vi "module-05-exercise-5-2.vi"() -> ()   [LabVIEW 2019]
uses:
  <vilib>/Rock Robotics/WPI/ThirdParty/JAS_Junk/TrajLib/Trajectory_Library.lvlib
panel:
  in  "Battery Voltage":dbl=10.0 min=0.0 max=14.0 step=0.1
  in  "Driver Shoot Disc Button":bool
  in  "Sensor - Have Disc to Shoot":bool
  out "Shooting In Progress":bool
  out "Digital State Chart":cluster{dbl, dbl, dbl, dbl, dbl, dbl}(graph)
  out "Ready to Shoot Disc":bool
  out "Shooting Motor Cmd On\n(Using splie for on/off Motor control)":bool
  out "Solenoid Engaged\n(Single solenoid)":bool
  out "Cur Time":dbl format="%20.3f"
  in  "Cancel":bool
  # "Traning exercise 5-2 template\nFlying disc shooter"
  # "F1"
  # "F2"
  # "F3"
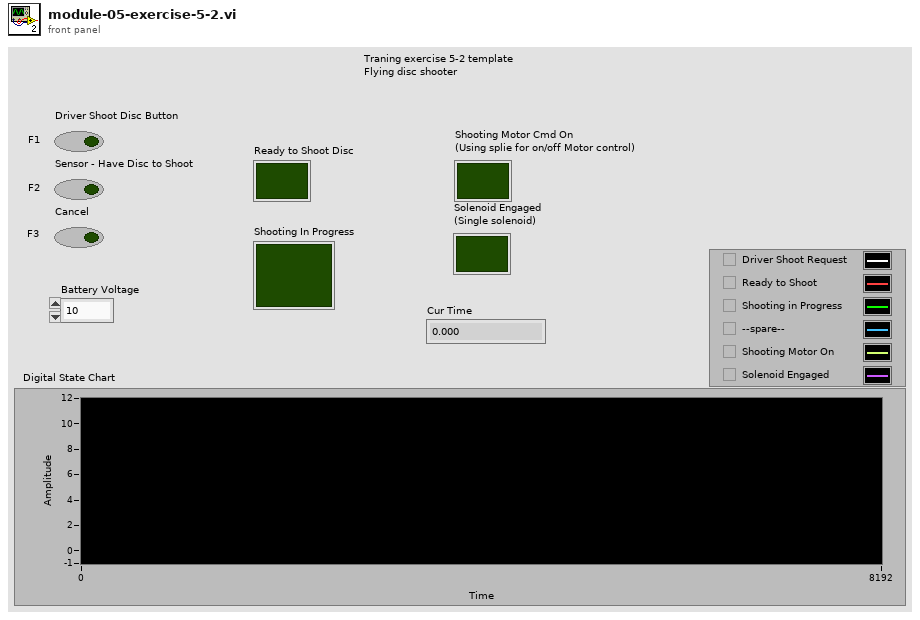
[diagram p1: front panel]
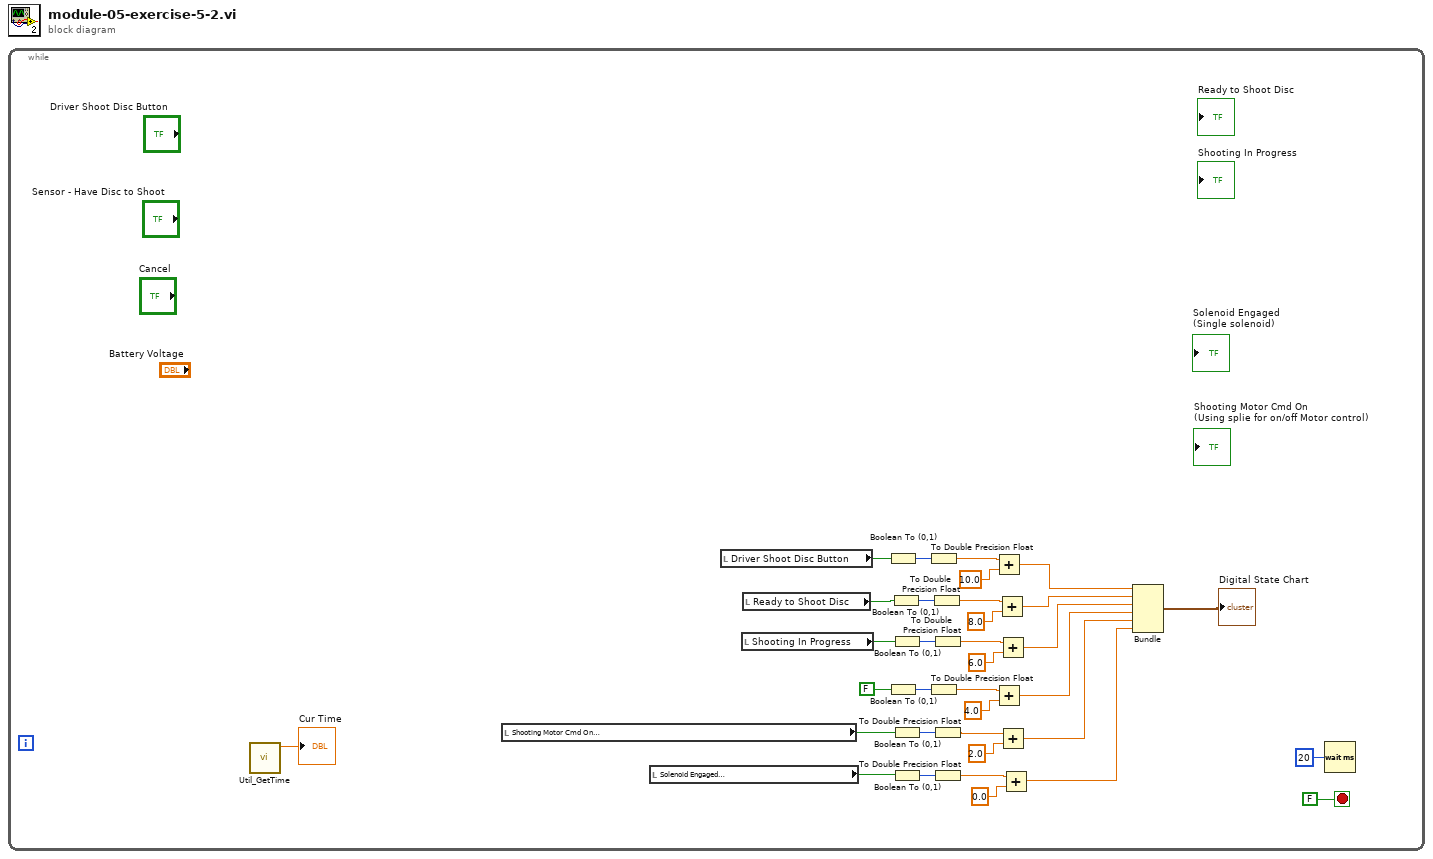
[diagram p0: block diagram]
diagram:
  n1 = while {
    stop <- FALSE stop-if-true
    n2 = call <vilib>:"Util_GetTime.vi"() -> ("FPGA_Time_Seconds"=→"Cur Time":dbl)  [unwired: 10 in, 1 out]
    n3 = local read "Shooting Motor Cmd On\n(Using splie for on/off Motor control)"() -> (w3:bool)
    n4 = local read "Solenoid Engaged\n(Single solenoid)"() -> (w7:bool)
    n5 = local read "Driver Shoot Disc Button"() -> (w8:bool)
    n6 = local read "Shooting In Progress"() -> (w1:bool)
    n7 = local read "Ready to Shoot Disc"() -> (w5:bool)
    n8 = Boolean To (0,1)(Boolean=w8) -> (0, 1=w32:i16)
    n9 = Boolean To (0,1)(Boolean=FALSE) -> (0, 1=w30:i16)
    n10 = Boolean To (0,1)(Boolean=w5) -> (0, 1=w27:i16)
    n11 = Boolean To (0,1)(Boolean=w1) -> (0, 1=w24:i16)
    n12 = Boolean To (0,1)(Boolean=w3) -> (0, 1=w21:i16)
    n13 = Boolean To (0,1)(Boolean=w7) -> (0, 1=w19:i16)
    n14 = To Double Precision Float(number=w32) -> (double precision float=w10:dbl)
    n15 = To Double Precision Float(number=w30) -> (double precision float=w29:dbl)
    n16 = To Double Precision Float(number=w27) -> (double precision float=w26:dbl)
    n17 = To Double Precision Float(number=w24) -> (double precision float=w23:dbl)
    n18 = To Double Precision Float(number=w21) -> (double precision float=w4:dbl)
    n19 = To Double Precision Float(number=w19) -> (double precision float=w18:dbl)
    n20 = Add(x=w10, y=10.0) -> (x+y=w9:dbl)
    n21 = Add(x=w29, y=4.0) -> (x+y=w13:dbl)
    n22 = Add(x=w26, y=8.0) -> (x+y=w15:dbl)
    n23 = Add(x=w23, y=6.0) -> (x+y=w14:dbl)
    n24 = Add(x=w4, y=2.0) -> (x+y=w17:dbl)
    n25 = Add(x=w18, y=0.0) -> (x+y=w16:dbl)
    n26 = Bundle(w9, w15, w14, w13, w17, w16) -> (→"Digital State Chart":cluster{dbl, dbl, dbl, dbl, dbl, dbl})  [unwired: 1 in]
    n27 = Wait (ms)(milliseconds to wait=u32 20) -> ()  [unwired: 1 out]
  }
